vi "待机状态数据存储写入和切换量程(子VI).vi"   [LabVIEW 2016, in "斯坦道CODMn.lvlib"]
uses:
  <vilib>/ptbypt/NI_PtbyPt.lvlib
types:
  T1 = cluster{"时间":timestamp, "测量模式":string, "数据类型":string, "检测值":sgl, "单位":string, "数据标识":string, "因子编码":string, "标样参考值":sgl, "ORP-A":sgl, "ORP-B":sgl, "ORP-K":sgl, "COD滴定值":sgl, "高锰酸钾滴定数":sgl, "温度":sgl, "量程":sgl, "LastTime":timestamp}
  T2 = cluster{"因子编码":u32, "单位":u16, "标样参考值":sgl, "水样数据时间":timestamp, "水样实测值":sgl, "水样数据标识":string, "标样数据时间":timestamp, "标样实测值":sgl, "标样数据标识":string, "空白数据时间":timestamp, "空白实测值":sgl, "空白数据标识":string, "零点核查数据时间":timestamp, "零点核查实测值":sgl, "零点核查数据标识":string, "跨度核查数据时间":timestamp, "跨度核查实测值":sgl, "跨度核查数据标识":string, "加标回收数据时间":timestamp, "加标回收实测值":sgl, "加标回收数据标识":string, "平行样数据时间":timestamp, "平行样实测值":sgl, "平行样数据标识":string}
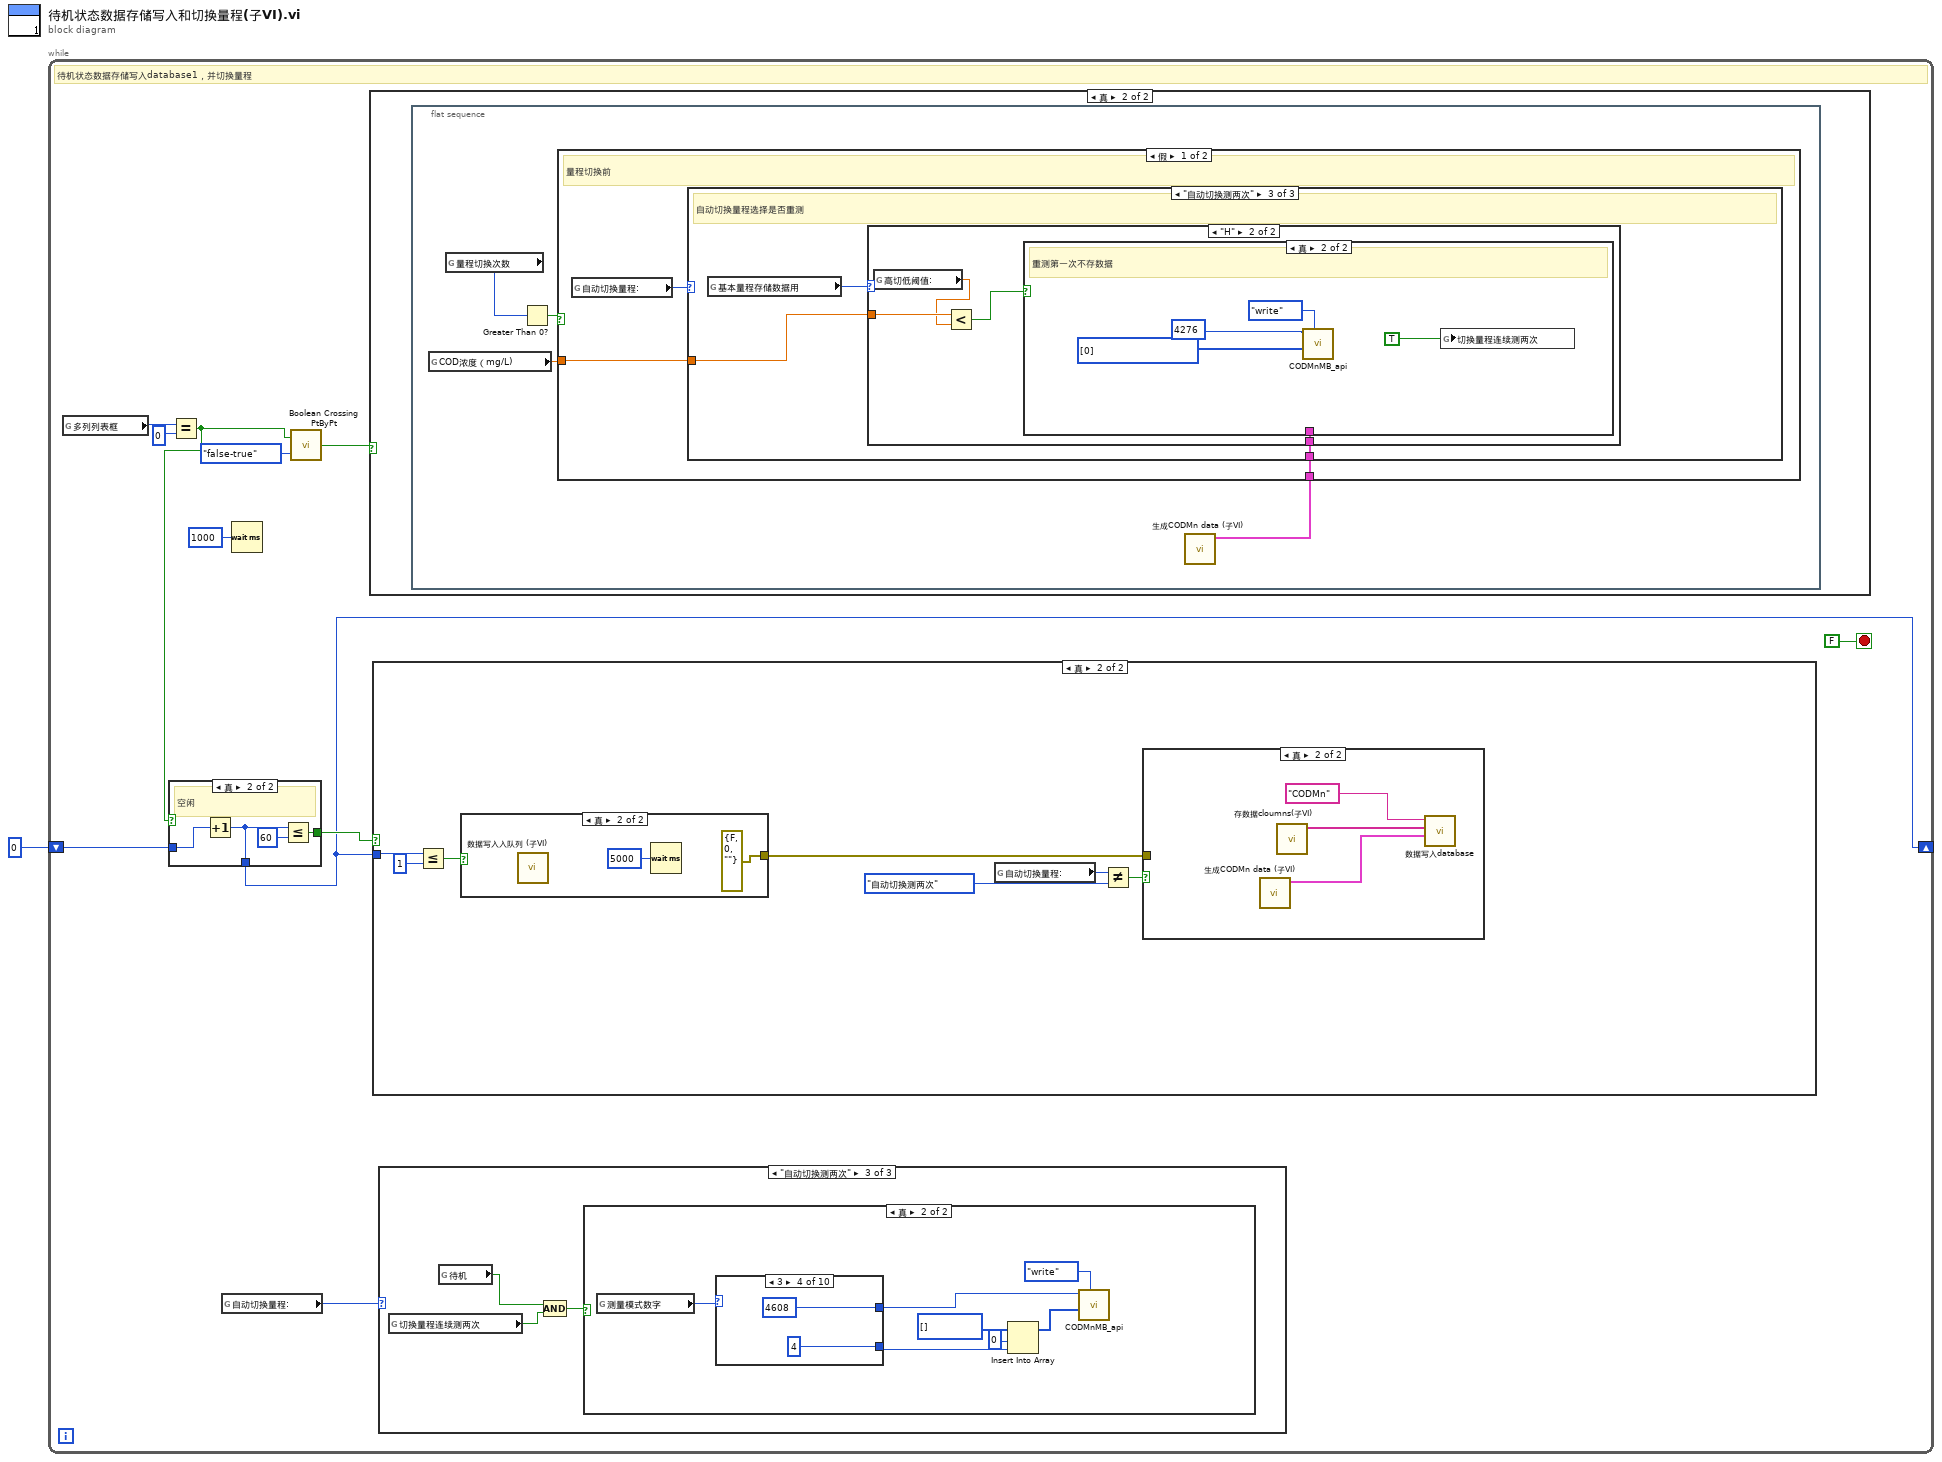
[diagram p0: block diagram]
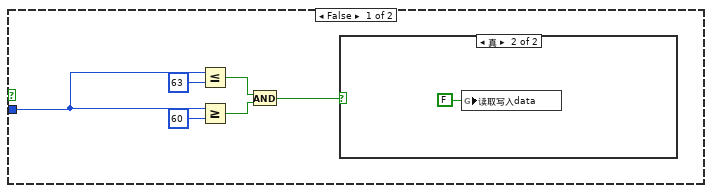
[diagram p2: hidden frame]
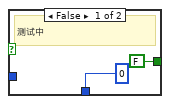
[diagram p6: hidden frame]
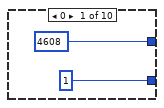
[diagram p10: hidden frame]
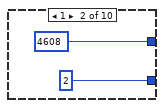
[diagram p11: hidden frame]
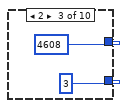
[diagram p12: hidden frame]
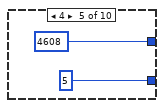
[diagram p13: hidden frame]
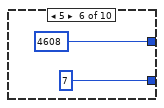
[diagram p14: hidden frame]
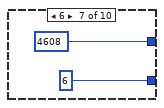
[diagram p15: hidden frame]
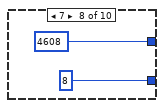
[diagram p16: hidden frame]
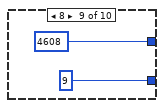
[diagram p17: hidden frame]
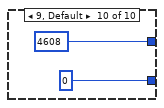
[diagram p18: hidden frame]
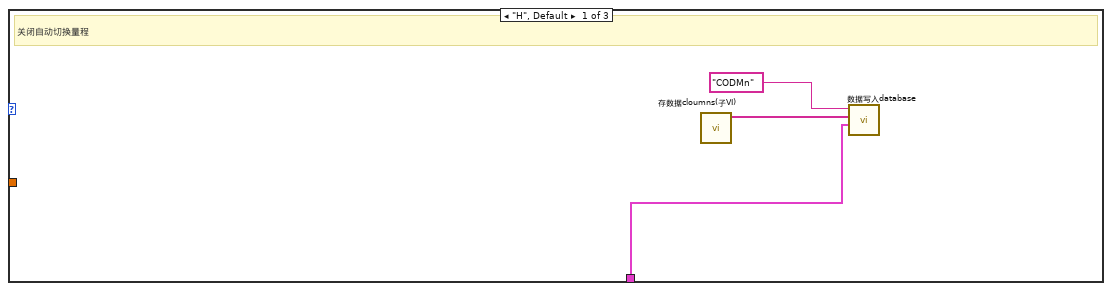
[diagram p20: hidden frame]
diagram:
  n1 = while {
    shift-right: [w2] -> _
    shift-left: 0 ("y") -> [w7]
    stop <- FALSE stop-if-true
    # "待机状态数据存储写入database1，并切换量程"
    n2 = global read "运行时序全局变量.vi" "多列列表框"() -> (w9:i32)
    n3 = Equal?(x=w9, y=0) -> (x = y?=w4:bool)
    n4 = case shown="真" w4 {
      tunnel: w7 -> [_ w36]
      tunnel: [0 w35] -> w2
      tunnel: [FALSE w34] -> w5
      frame False {
        # "测试中"
      }
      frame True {
        # "空闲"
        n5 = Increment(x=w36) -> (x+1=w35:i32)
        n6 = Less Or Equal?(x=w35, y=u32 60) -> (x <= y?=w34:bool)
      }
    }
    n7 = global read "CODMn断电保存全局变量.vi" "自动切换量程:"() -> (w8:enum16{"L", "H", "自动切换测一次", "自动切换测两次"})
    n8 = Wait (ms)(milliseconds to wait=u32 1000 ("等待时间（毫秒）")) -> ()  [unwired: 1 out]
    n9 = call <vilib>:"Boolean Crossing PtByPt.vi"("direction"=enum16{"either", "false-true", "true-false"}."false-true", "input"=w4) -> ("crossing"=w3:bool)  [unwired: 1 in]
    n10 = case shown="真" w3 {
      frame False {
      }
      frame True {
        n11 = flat-sequence {
          frame #0 {
            n12 = global read "COD浓度全局变量.vi" "COD浓度（mg/L)"() -> (w69:dbl)
            n13 = global read "COD内部交互全局.vi" "量程切换次数"() -> (w68:u8)
            n14 = Greater Than 0?(x=w68) -> (x > 0?=w70:bool)
            n15 = call "生成CODMn data (子VI).vi"() -> ("data"=w71:T1)  [unwired: 11 in]
            n16 = case shown="假" w70 {
              tunnel: w71 -> [w74 w132]
              tunnel: w69 -> [w73 _]
              frame False {
                # "量程切换前"
                n17 = global read "CODMn断电保存全局变量.vi" "自动切换量程:"() -> (w72:enum16{"L", "H", "自动切换测一次", "自动切换测两次"})
                n18 = case shown="\"自动切换测两次\"" w72 {
                  tunnel: w74 -> [w75 w80 w106]
                  tunnel: w73 -> [_ w79 w105]
                  frame "H", Default {
                    # "关闭自动切换量程"
                    n19 = call "存数据cloumns(子VI).vi"() -> ("数组"=w77:string[])  [unwired: 11 in]
                    n20 = call "数据写入database.vi"("data"=w75, "columns"=w77, "table"="CODMn") -> ()  [unwired: 8 in, 1 out]
                  }
                  frame "自动切换测一次" {
                    # "自动切换量程选择是否重测"
                    n21 = global read "COD内部交互全局.vi" "基本量程存储数据用"() -> (w78:enum16{"L", "H", "AUTO"})
                    n22 = global read "COD测量模式全局.vi" "测量模式"() -> (w86:string)
                    n23 = Not Equal?(x=w86, y="水样测试") -> (x != y?=w84:bool)
                    n24 = case shown="真" w84 {
                      tunnel: [w101 w102] -> w83
                      tunnel: w79 -> [w101 _]
                      frame False {
                      }
                      frame True {
                        n25 = global read "CODMn断电保存全局变量.vi" "测量数据区"() -> (w103:T2)
                        n26 = Unbundle By Name(w103) -> ("水样实测值"=w102:sgl)
                      }
                    }
                    n27 = case shown="\"H\"" w78 {
                      tunnel: w83 -> [w90 w96]
                      frame "L", Default {
                        n28 = global read "COD内部交互全局.vi" "高锰酸钾报警"() -> (w87:bool)
                        n29 = global read "CODMn断电保存全局变量.vi" "低切高阈值:"() -> (w88:dbl)
                        n30 = Greater?(x=w90, y=w88) -> (0:w91:bool)
                        n31 = Or(x=w87, y=w91) -> (x .or. y?=w89:bool)
                        n32 = case shown="真" w89 {
                          frame False {
                          }
                          frame True {
                            n33 = call "CODMnMB_api.vi"("STEP"=enum16{"open", "read", "write", "close"}."write", "values"=u16[] [1], "starting address"=u16 4276) -> ()  [unwired: 6 in, 3 out]
                          }
                        }
                      }
                      frame "H" {
                        n34 = global read "CODMn断电保存全局变量.vi" "高切低阈值:"() -> (w95:dbl)
                        n35 = Less?(x=w96, y=w95) -> (x < y?=w97:bool)
                        n36 = case shown="真" w97 {
                          frame False {
                          }
                          frame True {
                            n37 = call "CODMnMB_api.vi"("STEP"=enum16{"open", "read", "write", "close"}."write", "values"=u16[] [0], "starting address"=u16 4276) -> ()  [unwired: 6 in, 3 out]
                          }
                        }
                      }
                    }
                    n38 = call "存数据cloumns(子VI).vi"() -> ("数组"=w82:string[])  [unwired: 11 in]
                    n39 = call "数据写入database.vi"("data"=w80, "columns"=w82, "table"="CODMn") -> ()  [unwired: 8 in, 1 out]
                  }
                  frame "自动切换测两次" {
                    # "自动切换量程选择是否重测"
                    n40 = global read "COD内部交互全局.vi" "基本量程存储数据用"() -> (w104:enum16{"L", "H", "AUTO"})
                    n41 = case shown="\"H\"" w104 {
                      tunnel: w105 -> [w111 w122]
                      tunnel: w106 -> [w110 w121]
                      frame "L", Default {
                        n42 = global read "CODMn断电保存全局变量.vi" "低切高阈值:"() -> (w108:dbl)
                        n43 = global read "COD内部交互全局.vi" "高锰酸钾报警"() -> (w107:bool)
                        n44 = Greater?(x=w111, y=w108) -> (0:w112:bool)
                        n45 = Or(x=w112, y=w107) -> (x .or. y?=w109:bool)
                        n46 = case shown="真" w109 {
                          tunnel: w110 -> [w113 _]
                          frame False {
                            n47 = call "存数据cloumns(子VI).vi"() -> ("数组"=w115:string[])  [unwired: 11 in]
                            n48 = global write "COD内部交互全局.vi" "data"(w113) -> ()
                            n49 = call "数据写入database.vi"("data"=w113, "columns"=w115, "table"="CODMn") -> ()  [unwired: 8 in, 1 out]
                          }
                          frame True {
                            n50 = global write "COD内部交互全局.vi" "切换量程连续测两次"(TRUE ("切换量程连续测两次")) -> ()
                            n51 = call "CODMnMB_api.vi"("STEP"=enum16{"open", "read", "write", "close"}."write", "values"=u16[] [1], "starting address"=u16 4276) -> ()  [unwired: 6 in, 3 out]
                          }
                        }
                      }
                      frame "H" {
                        n52 = global read "CODMn断电保存全局变量.vi" "高切低阈值:"() -> (w120:dbl)
                        n53 = Less?(x=w122, y=w120) -> (x < y?=w123:bool)
                        n54 = case shown="真" w123 {
                          tunnel: w121 -> [w124 _]
                          frame False {
                            n55 = call "存数据cloumns(子VI).vi"() -> ("数组"=w126:string[])  [unwired: 11 in]
                            n56 = call "数据写入database.vi"("data"=w124, "columns"=w126, "table"="CODMn") -> ()  [unwired: 8 in, 1 out]
                          }
                          frame True {
                            # "重测第一次不存数据"
                            n57 = call "CODMnMB_api.vi"("STEP"=enum16{"open", "read", "write", "close"}."write", "values"=u16[] [0], "starting address"=u16 4276) -> ()  [unwired: 6 in, 3 out]
                            n58 = global write "COD内部交互全局.vi" "切换量程连续测两次"(TRUE ("切换量程连续测两次")) -> ()
                          }
                        }
                      }
                    }
                  }
                }
              }
              frame True {
                # "防止无限切量程"
                n59 = global write "COD内部交互全局.vi" "量程切换次数"(u8 0 ("量程切换次数")) -> ()
                n60 = call "存数据cloumns(子VI).vi"() -> ("数组"=w134:string[])  [unwired: 11 in]
                n61 = call "数据写入database.vi"("data"=w132, "columns"=w134, "table"="CODMn") -> ()  [unwired: 8 in, 1 out]
              }
            }
          }
        }
      }
    }
    n62 = case shown="真" w5 {
      tunnel: w2 -> [w15 w23]
      frame False {
        n63 = Less Or Equal?(x=w15, y=63) -> (x <= y?=w18:bool)
        n64 = Greater Or Equal?(x=w15, y=60) -> (x >= y?=w17:bool)
        n65 = And(x=w18, y=w17) -> (x .and. y?=w13:bool)
        n66 = case shown="真" w13 {
          frame False {
          }
          frame True {
            n67 = global write "COD内部交互全局.vi" "读取写入data"(FALSE ("读取写入data")) -> ()
          }
        }
      }
      frame True {
        n68 = Less Or Equal?(x=w23, y=1) -> (x <= y?=w21:bool)
        n69 = case shown="真" w21 {
          tunnel: [_ errorcluster {"status"=FALSE, "code"=0, "source"=""} ("错误常量")] -> w20
          frame False {
          }
          frame True {
            n70 = call "数据写入入队列 (子VI).vi"() -> ()  [unwired: 12 in]
            n71 = Wait (ms)(milliseconds to wait=u32 5000 ("等待时间（毫秒）")) -> ()  [unwired: 1 out]
          }
        }
        n72 = global read "CODMn断电保存全局变量.vi" "自动切换量程:"() -> (w26:enum16{"L", "H", "自动切换测一次", "自动切换测两次"})
        n73 = Not Equal?(x=w26, y=enum16{"L", "H", "自动切换测一次", "自动切换测两次"}."自动切换测两次") -> (x != y?=w25:bool)
        n74 = case shown="真" w25 {
          tunnel: w20 -> [_ _]
          frame False {
          }
          frame True {
            n75 = call "生成CODMn data (子VI).vi"() -> ("data"=w31:T1)  [unwired: 11 in]
            n76 = call "存数据cloumns(子VI).vi"() -> ("数组"=w30:string[])  [unwired: 11 in]
            n77 = call "数据写入database.vi"("data"=w31, "columns"=w30, "table"="CODMn") -> ()  [unwired: 8 in, 1 out]
          }
        }
      }
    }
    n78 = case shown="\"自动切换测两次\"" w8 {
      frame "H", Default {
      }
      frame "自动切换测一次" {
      }
      frame "自动切换测两次" {
        n79 = global read "COD内部交互全局.vi" "切换量程连续测两次"() -> (w39:bool)
        n80 = global read "COD内部交互全局.vi" "待机"() -> (w38:bool)
        n81 = Compound Arithmetic op=AND ("复合运算")(w38, w39) -> (w40:bool)
        n82 = case shown="真" w40 {
          frame False {
          }
          frame True {
            n83 = global read "COD内部交互全局.vi" "测量模式数字"() -> (w41:i32)
            n84 = case shown="3" w41 {
              tunnel: [u16 4608 ("address") u16 4608 ("address") u16 4608 ("address") u16 4608 ("address") u16 4608 ("address") u16 4608 ("address") u16 4608 ("address") u16 4608 ("address") u16 4608 ("address") u16 4608 ("address")] -> w42
              tunnel: [u16 1 ("address") u16 2 ("address") u16 3 ("address") u16 4 ("address") u16 5 ("address") u16 7 ("address") u16 6 ("address") u16 8 ("address") u16 9 ("address") u16 0 ("address")] -> w47
              frame 0 {
              }
              frame 1 {
              }
              frame 2 {
              }
              frame 3 {
              }
              frame 4 {
              }
              frame 5 {
              }
              frame 6 {
              }
              frame 7 {
              }
              frame 8 {
              }
              frame 9, Default {
              }
            }
            n85 = Insert Into Array(array=u16[] [] ("values"), index=0 ("索引"), new element=w47) -> (w43:u16[])
            n86 = call "CODMnMB_api.vi"("STEP"=enum16{"open", "read", "write", "close"}."write", "values"=w43, "starting address"=w42) -> ()  [unwired: 6 in, 3 out]
          }
        }
      }
    }
  }
